vi "FPGA_main.vi"() -> ()   [LabVIEW 2025]
uses:
  <vilib>/Platform/TimedLoop/XDataNode/timing_clust.ctl
  <vilib>/Platform/TimedLoop/XDataNode/nitl_modes.ctl
  <vilib>/Platform/TimedLoop/XDataNode/wakeup.ctl
  <vilib>/rvi/Emulation/niFpgaGetClockAttributes.vi
  <vilib>/rvi/Emulation/niFpgaSctlEmulationGetInTimedLoop.vi
  <vilib>/rvi/Emulation/niFpgaEmulationReportErrorSimple.vi
  <vilib>/rvi/DataTransferAndStorage/Container/Common/niFpgaContainerGetUniqueNameForEmu.vi
  <vilib>/rvi/DataTransferAndStorage/Container/Common/niFpgaContainerSetEmuInfo.vi
  <vilib>/rvi/eio/common/nirviEmuReportErrorAndStop.vi
  <vilib>/rvi/DataTransferAndStorage/Container/Common/niFpgaContainerExecOnDevCompGetState.vi
  <vilib>/rvi/Emulation/niFpgaEmulationIsFPGAContextNoSignature.vi
  <vilib>/rvi/errors/niFpgaSetErrorForExecOnDevCompSimple.vi
  <vilib>/rvi/FIFO/Fifo_Resource/nirvififoEmulationSetSize.vi
  <vilib>/rvi/FIFO/Fifo_Resource/nirviFifoEmulationQueueMgr.vi
  <instcachedir>/0/nirviFifoEmulationQueueMgr_E5CAEC123FF24DC58D834DCA3CDAA9B5.lvgen/nirviFifoEmulationQueueMgr_E5CAEC123FF24DC58D834DCA3CDAA9B5_002.vi
  <vilib>/rvi/FIFO/Fifo_Resource/nirvififoEmulationDetermineInputValidOut.vi
  <vilib>/rvi/FIFO/Fifo_Resource/nirvififoEmulationCreateLock.vi
  <vilib>/rvi/Emulation/niFpgaProcessEmulError.vi
  <vilib>/rvi/FIFO/Fifo_Resource/nirvififoEmulationObtainLock.vi
  <vilib>/rvi/FIFO/Fifo_Resource/nirvififoEmulationReleaseLock.vi
  <vilib>/rvi/occurrence/nirviWaitOnOccurrenceBase.vi
  <vilib>/rvi/errors/nirviReportUnexpectedCaseInternalError.vi
  <vilib>/rvi/errors/nirviReportUnexpectedCaseInternalError (U32).vi
  <vilib>/Utility/error.llb/Clear Errors.vi
  <vilib>/eio/utilities/niEioResolveVilibRelativePath.vi
  <vilib>/rvi/interface/RandomDataEmulation/niFpgaRandomDataHandleErrors.vi
  <vilib>/rvi/Emulation/niFpgaCriticalErrorInLSC.vi
  <vilib>/rvi/eio/common/nirviEmuTemplateMethod_errors.vi
  <vilib>/rvi/LocalResourceManager/LocalResourceManager.xnode
  <vilib>/rvi/DataTransferAndStorage/Container/XNode/niFpgaContainer.xnode
  <vilib>/rvi/FIFO/Fifo_Resource/niFpgaFifoEmulationRefIn.vi
  <vilib>/Platform/TimedLoop/XDataNode/XDataNode.xnode
  <vilib>/eio/EIONode/EIONode.xnode
  <vilib>/Platform/TimedLoop/XDataNode/XDNodeRunTimeDep.lvlib
panel:
  in  "hightimes":i32[](array[numeric])=[0, 0, 0]
  out "buttons":u64
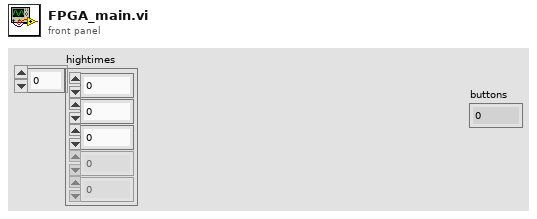
[diagram p1: front panel]
types:
  T1 = typedef "XDNodeRunTimeDep.lvlib/timing_clust.ctl" = cluster{"Expected End [f-1]":u64, "Actual End [f-1]":u64, "Finished Late? [f-1]":bool, "Expected End [i-1]":u64, "Actual End [i-1]":u64, "Finished Late? [i-1]":bool, "Expected Start [i]":u64, "Actual Start [i]":u64, "Expected Start [f]":u64, "Actual Start [f]":u64, "Source Name":string, "Structure Name":string, "Period":i64, "Deadline":i64, "Offset":i64, "Start":i64, "Priority":i32, "Timeout":i32, "Mode":T2, "Wakeup Reason":T3, "Error":errorcluster, "Source Type":string, "Secondary Source Type":string, "Global End Time":u64, "Global Start Time":u64, "Frame Duration":u64, "Iteration Duration":u64, "Assigned CPU":i32, "I/O Scan Engine Mode":u32}
  T2 = typedef "XDNodeRunTimeDep.lvlib/nitl_modes.ctl" = enum32{"No Change", "Process missed periods, maintain original phase", "Discard missed periods, maintain original phase", "Process missed periods, ignore original phase", "Discard missed periods, ignore original phase"}
  T3 = typedef "XDNodeRunTimeDep.lvlib/wakeup.ctl" = enum32{"Normal", "Aborted", "Asynchronous wakeup", "Timing source error", "Timed loop error", "Timeout"}
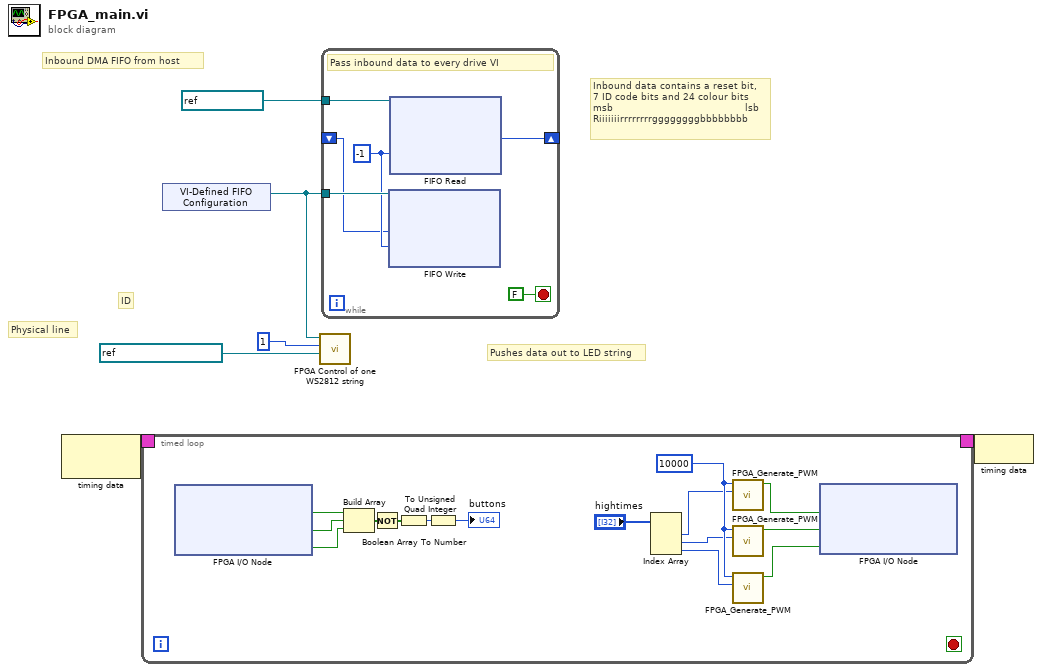
[diagram p0: block diagram]
diagram:
  # "Inbound DMA FIFO from host"
  # "Pushes data out to LED string"
  # "Physical line"
  # "ID"
  # "Inbound data contains a reset bit,\n7 ID code bits and 24 colour bits\nmsb                                            lsb\nRiiiiiiirrrrrrrrggggggggbbbbbbbb"
  n1 = node-c288() -> (w2:T1)  [unwired: 1 in]
  n2 = timed-loop {
    timing: w2 -> [_]
    timing-out: [_] -> w1
    stop <- _ stop-if-true
    w18 = 10000 ("period(ticks)")
    n3 = xnode "FPGA I/O Node"() -> ("ConnectorB/DIO0"=w17:bool, "ConnectorB/DIO1"=w16:bool, "ConnectorB/DIO2"=w15:bool)  [unwired: 3 in, 3 out]
    n4 = Build Array(w17, w16, w15) -> (w14:bool[])
    n5 = Not(x=w14) -> (.not. x?=w7:bool[])
    n6 = Boolean Array To Number(Boolean array=w7) -> (number=w13:u8)
    n7 = To Unsigned Quad Integer(1:w13) -> (0:→"buttons":u64)
    n8 = Index Array(array="hightimes") -> (element #1=w10:i32, element #2=w9:i32, element #3=w8:i32)  [unwired: 3 in]
    n9 = call "FPGA_Generate_PWM.vi"("high-time (ticks)"=w10, "period(ticks)"=w18) -> ("PWM out"=w21:bool)  [unwired: 9 in]
    n10 = call "FPGA_Generate_PWM.vi"("high-time (ticks)"=w9, "period(ticks)"=w18) -> ("PWM out"=w20:bool)  [unwired: 9 in]
    n11 = call "FPGA_Generate_PWM.vi"("high-time (ticks)"=w8, "period(ticks)"=w18) -> ("PWM out"=w19:bool)  [unwired: 9 in]
    n12 = xnode "FPGA I/O Node"("ConnectorB/DIO3"=w21, "ConnectorB/DIO4"=w20, "ConnectorB/DIO5"=w19) -> ()  [unwired: 3 in, 3 out]
  }
  n13 = xnode "VI-Defined FIFO Configuration"() -> ("FIFO Out"=w3:refnum<k21>)
  n14 = call "FPGA Control of one WS2812 string.vi"("FPGA DO line"=refnum<k21> "ConnectorA/DIO0" ("FPGA I/O In"), "Wire ID"=u8 1 ("ID"), "FIFO In"=w3) -> ()  [unwired: 9 in]
  n15 = while {
    tunnel: refnum<k21> "DMA FIFO" ("FIFO In") -> [w29]
    tunnel: w3 -> [w27]
    shift-right: [w25] -> _
    shift-left: _ -> [w24]
    stop <- FALSE stop-if-true
    w26 = -1 ("Timeout")
    # "Pass inbound data to every drive VI"
    n16 = xnode ("FIFO Write")("Element"=w24, "Timeout"=w26, "FIFO In"=w27) -> ()  [unwired: 2 out]
    n17 = xnode ("FIFO Read")("Timeout"=w26, "FIFO In"=w29) -> ("Element"=w25:u32)  [unwired: 2 out]
  }
  n18 = node-c288(w1) -> ()
